vi "EncodeMaskedBytes.vi"(8 "error in (no error)":errorcluster, 11 "Raw Data":string) -> (0 "error out":errorcluster, 3 "Encoded Data":string)   [LabVIEW 2014, in "QwaveSys RPi Training Library.lvlib" / "WebSockets.lvlib"]
doc: "Unmasks incoming data. Data sent to the client does not need to be masked.\nWebSockets API 1.3.0.13\nSam Sharp - Intelligent Energy\nCopyright (c) 2015, Intelligent Energy"
uses:
  <vilib>/Q-Wave Systems/QwaveSys RPi Training Package (Demo)/Addons/WebSockets API/WebSockets/WebSockets.lvlib
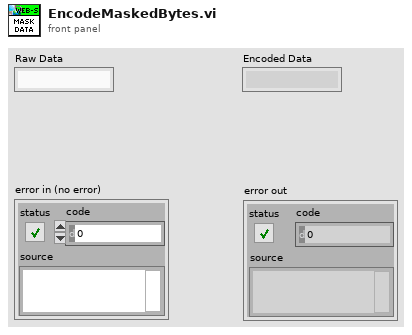
[diagram p1: front panel]
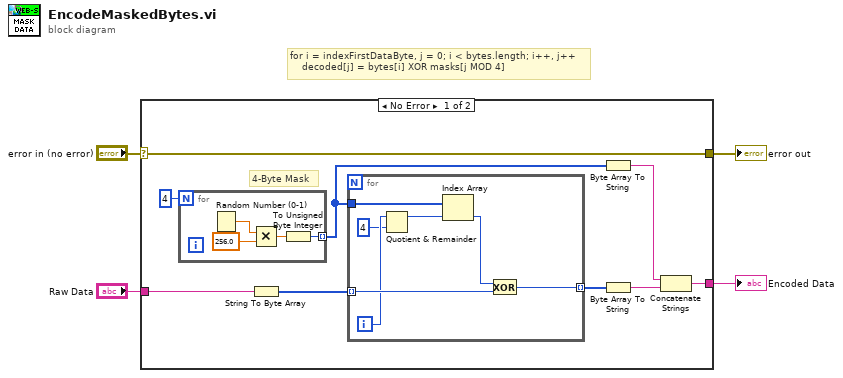
[diagram p0: block diagram]
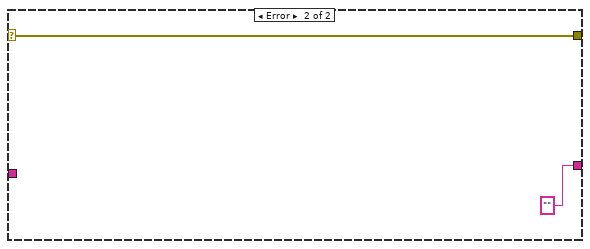
[diagram p2: hidden frame]
diagram:
  # "for i = indexFirstDataByte, j = 0; i < bytes.length; i++, j++\n    decoded[j] = bytes[i] XOR masks[j MOD 4]"
  n1 = case shown="No Error" "error in (no error)" {
    selector: "error in (no error)" -> [w13 w26]
    tunnel: "Raw Data" -> [w12 _]
    tunnel: [w5 "" ("Mask Bytes")] -> w4
    tunnel: [w13 w26] -> w1
    frame No Error {
      # "4-Byte Mask"
      n2 = for {
        N: 4 -> [_]
        tunnel: [w14] -> w8 mode=indexing
        n3 = Random Number (0-1)() -> (number: 0 to 1=w17:dbl)
        n4 = Multiply(x=w17, y=256.0) -> (x*y=w15:dbl)
        n5 = To Unsigned Byte Integer(number=w15) -> (unsigned 8bit integer=w14:u8)
      }
      n6 = String To Byte Array(string=w12) -> (unsigned byte array=w11:u8[])
      n7 = for {
        tunnel: w11 -> [w24] mode=indexing
        tunnel: w8 -> [w20]
        tunnel: [w18] -> w10 mode=indexing
        i -> [w23]
        n8 = Quotient & Remainder(x=w23, y=4) -> (x-y*floor(x/y)=w21:i32)  [unwired: 1 out]
        n9 = Index Array(array=w20, index=w21) -> (element=w19:u8)
        n10 = Exclusive Or(1:w24, 2:w19) -> (0:w18:u8)
      }
      n11 = Byte Array To String(unsigned byte array=w8) -> (string=w7:string)
      n12 = Byte Array To String(unsigned byte array=w10) -> (string=w6:string)
      n13 = Concatenate Strings(w7, w6) -> (w5:string)
    }
    frame Error {
    }
  }
  "Encoded Data" <- w4
  "error out" <- w1
